vi "Create Display Properties Update Object.vi"(4 "error in (no error)":errorcluster, 7 "Control in":refnum<vi>) -> (0 "error out":errorcluster, 3 "Font Settting out":refnum<class "Display Properties.lvclass">)   [LabVIEW 2015, in "Display Properties Manager.lvlib" / "Display Properties.lvclass"]
uses:
  Display Properties.lvclass
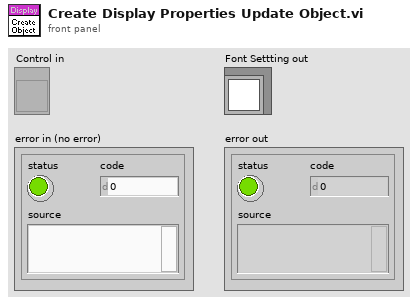
[diagram p1: front panel]
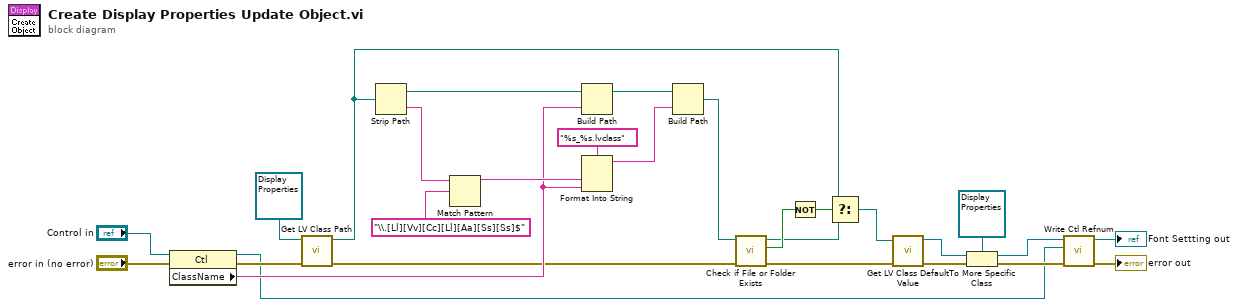
[diagram p0: block diagram]
diagram:
  n1 = property class="Ctl"(reference="Control in", error in="error in (no error)") -> (reference out=w1:refnum<vi>, error out=w25:errorcluster, "ClassName"=w19:string)
  n2 = call <vilib>:"Get LV Class Path.vi"("error in (no error)"=w25, "object"=refnum<class "Display Properties.lvclass"> refnum ("Runtime Font Manager.lvlib:Font Settting.lvclass")) -> ("error out"=w16:errorcluster, "class path"=w15:path)  [unwired: 8 in]
  n3 = Strip Path(path=w15) -> (stripped path=w24:path, name=w22:string)
  n4 = Match Pattern(string=w22, regular expression="\\.[Ll][Vv][Cc][Ll][Aa][Ss][Ss]$") -> (before substring=w20:string)  [unwired: 1 in, 3 out]
  n5 = Build Path(base path=w24, name or relative path=w19) -> (appended path=w23:path)
  n6 = Format Into String(format string="%s_%s.lvclass", w20, w19) -> (resulting string=w17:string)  [unwired: 2 in, 1 out]
  n7 = Build Path(base path=w23, name or relative path=w17) -> (appended path=w13:path)
  n8 = call <vilib>:"Check if File or Folder Exists.vi"("error in (no error)"=w16, "path"=w13) -> ("error out"=w9:errorcluster, "file or folder exists?"=w14:bool, "dup path"=w12:path)  [unwired: 7 in]
  n9 = Not(x=w14) -> (.not. x?=w11:bool)
  n10 = Select(t=w15, s=w11, f=w12) -> (s? t:f=w10:path)
  n11 = call <vilib>:"Get LV Class Default Value.vi"("error in (no error)"=w9, "class path"=w10) -> ("error out"=w8:errorcluster, "object"=w7:refnum<class>)  [unwired: 8 in]
  n12 = To More Specific Class(target class=refnum<class "Display Properties.lvclass"> refnum ("Runtime Font Manager.lvlib:Font Settting.lvclass"), reference=w7, error in=w8) -> (specific class reference=w5:refnum<class "Display Properties.lvclass">, error out=w3:errorcluster)
  n13 = call-dynamic "Write Ctl Refnum.vi"("Error In"=w3, "Ctl Refnum"=w1, "Font Settting in"=w5) -> ("Error Out"=→"error out":errorcluster, "Font Settting out"=→"Font Settting out":refnum<class "Display Properties.lvclass">)  [unwired: 3 in]
